vi "123test.vi"() -> ()   [LabVIEW 2023]
panel:
  out "XY 그래프":cluster{i32[], dbl[]}(graph)
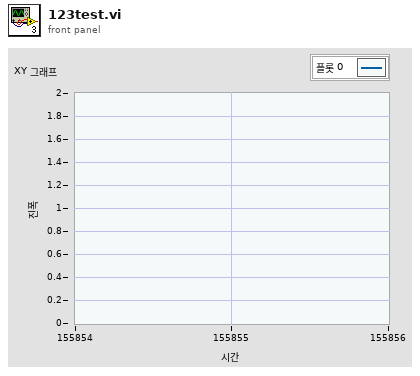
[diagram p1: front panel]
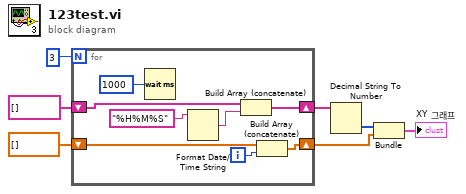
[diagram p0: block diagram]
diagram:
  n1 = for {
    N: 3 -> [_]
    shift-right: [w12] -> w2
    shift-left: dbl[] [] -> [w13]
    shift-right: [w8] -> w4
    shift-left: string[] [] -> [w10]
    i -> [w11]
    n2 = Wait (ms)(milliseconds to wait=u32 1000 ("대기 시간 (ms)")) -> ()  [unwired: 1 out]
    n3 = Format Date/Time String(time format string (%c)="%H%M%S" ("시간 포맷 문자열 (%c)")) -> (date/time string=w9:string)  [unwired: 2 in]
    n4 = Build Array (concatenate)(w10, w9) -> (w8:string[])
    n5 = Build Array (concatenate)(w13, w11) -> (w12:dbl[])
  }
  n6 = Decimal String To Number(string=w4) -> (number=w3:i32[])  [unwired: 2 in, 1 out]
  n7 = Bundle(w3, w2) -> (→"XY 그래프":cluster{i32[], dbl[]})  [unwired: 1 in]
